vi "Seriell-ECD.vi"(0 "FPGA-VI-Referenz":refnum<k20>, 1 "SPvorgebenMod2":string[](array[string])=[":0622010121", ":0621010121", ":0626010121", ":0620010121", ":0624010121", ":0625010121", ":0623010121"], 5 "MWabfragenMod2":string[](array[string])=[":06220401210120", ":06210401210120", ":06260401210120", ":06200401210120", ":06240401210120", ":06250401210120", ":06230401210120"], 9 "MWAntwortMod2":string[](array[string])=[":0622020121", ":0621020121", ":0626020121", ":0620020121", ":0624020121", ":0625020121", ":0623020121"], 11 "FaktorMod2":dbl[](array[numeric])=[0.00625, 0.00625, 0.15625, 0.00015625, 0.00625, 0.00625, 0.00015625], 12 "SPquittieren":string[](array[string])=[":0422000005", ":0421000005", ":0426000005", ":0420000005", ":0424000005", ":0425000005", ":0423000005"]) -> (4 "Fehler":errorcluster)   [LabVIEW 2017]
uses:
  GVRefStrom.vi
  GVHorstSP.vi
  GVMWHorst.vi
  gvbooleschRT.vi
  <vilib>/Utility/error.llb/Error Cluster From Error Code.vi
  <vilib>/rvi/errors/niLvFpgaAdjustHostInterfaceError.vi
  GVECDs.vi
  <vilib>/rvi/interface/nirviMethod/nirviMethod.xnode
  FPGA Bitfiles/HAGAR-VECD_FPGATarget_FPGA-ProgrammECD_WS++LmW9gGg.lvbitx
  FPGA-Programm_ECD.vi
  <vilib>/regexp/Match Regular Expression.xnode
  <vilib>/FPGAPlugInAG/cRIO-9035/niLvFpga_WriteFifo_cRIO-9035.vi
  <vilib>/rvi/errors/niLvFpgaMergeErrorWithErrorCode.vi
  <vilib>/FPGAPlugInAG/cRIO-9035/niLvFpga_ReadFifo_cRIO-9035.vi
panel:
  in  "Fehler":errorcluster caption="Fehler (Ausgang)"
  out "ECD2":string
  out "ECD1":string
  out "Fehler":bool[](array[boolean])
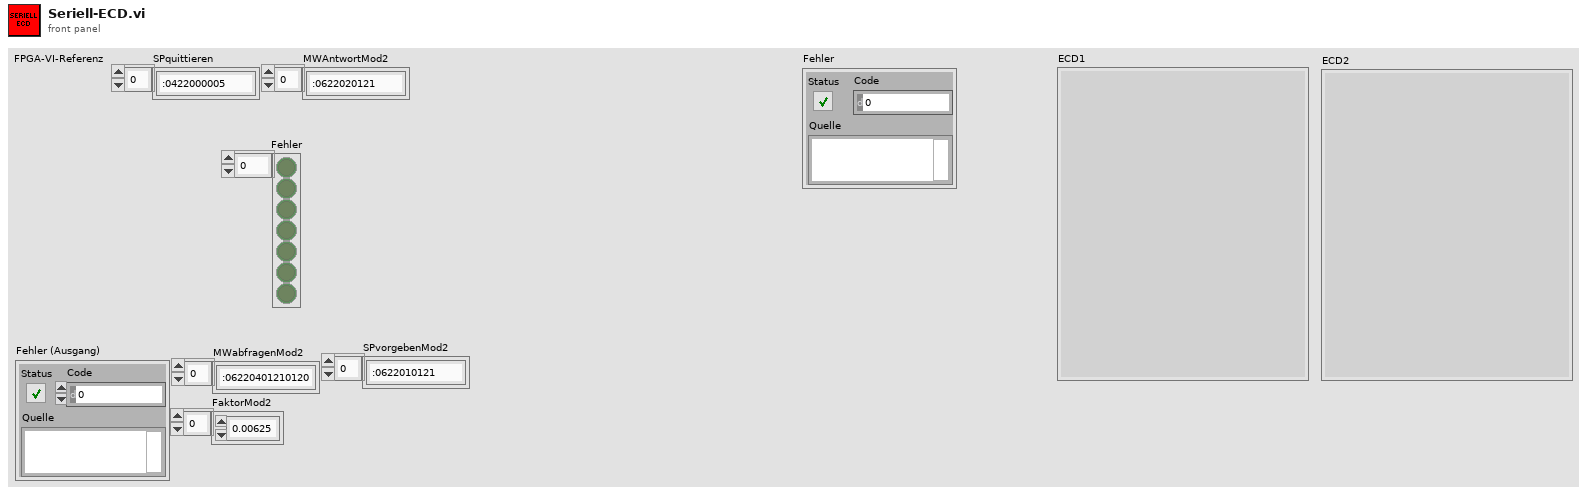
[diagram p1: front panel]
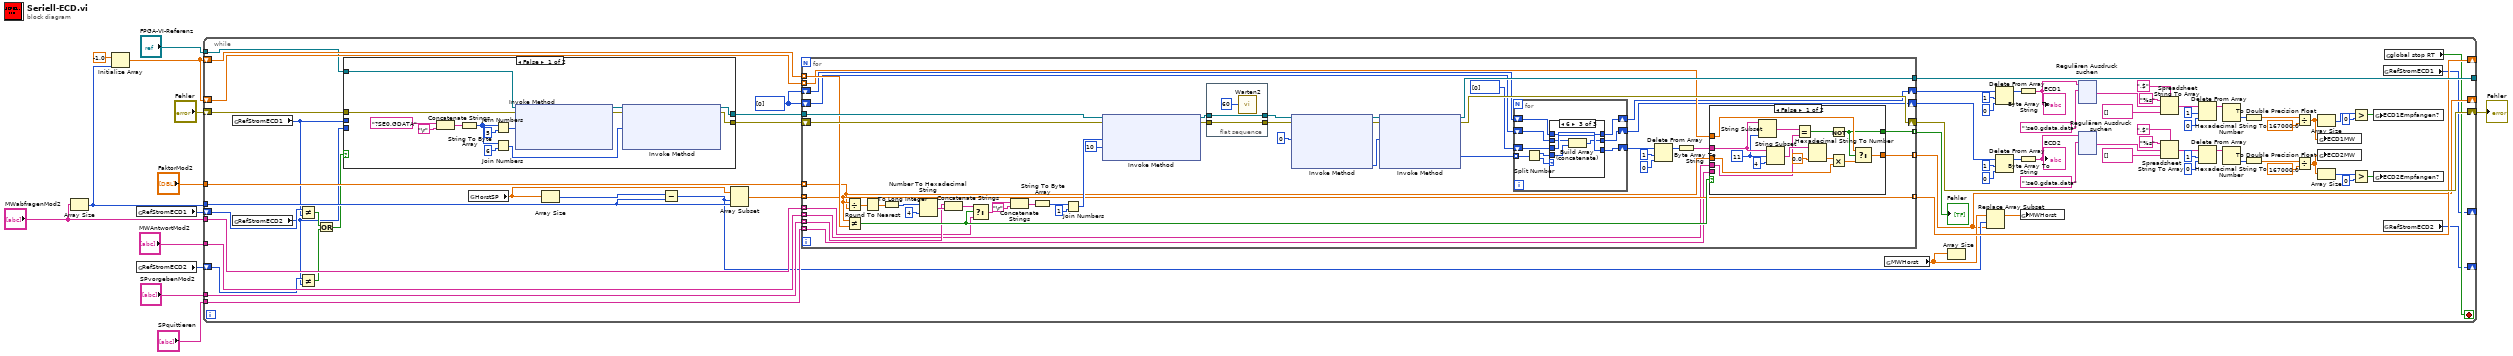
[diagram p0: block diagram]
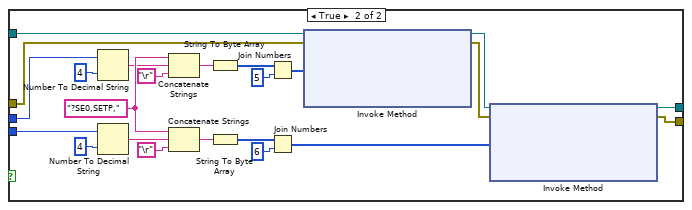
[diagram p2: hidden frame]
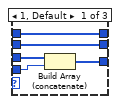
[diagram p3: hidden frame]
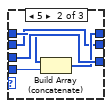
[diagram p4: hidden frame]
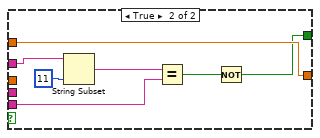
[diagram p5: hidden frame]
diagram:
  n1 = Array Size(array="MWabfragenMod2") -> (size(s)=w3:i32)
  n2 = Initialize Array(-1.0 ("Element"), w3) -> (w5:dbl[])
  n3 = global read "GVRefStrom.vi" "RefStromECD1"() -> (w2:i16)
  n4 = global read "GVRefStrom.vi" "RefStromECD2"() -> (w1:i16)
  n5 = while {
    shift-right: [w88] -> w4
    shift-left: "Fehler" -> [w68]
    shift-right: [w86] -> _
    shift-left: w5 -> [w87]
    shift-right: [w25] -> _
    shift-left: w5 -> [w84]
    tunnel: "SPvorgebenMod2" -> [w83]
    tunnel: "MWabfragenMod2" -> [w82]
    tunnel: "FaktorMod2" -> [w81]
    tunnel: "MWAntwortMod2" -> [w80]
    tunnel: "SPquittieren" -> [w79]
    tunnel: "FPGA-VI-Referenz" -> [w69]
    tunnel: [w89] -> _
    tunnel: w3 -> [w29]
    shift-right: [w22] -> _
    shift-left: w2 -> [w20]
    shift-right: [w21] -> _
    shift-left: w1 -> [w19]
    stop <- w23 stop-if-true
    w78 = u8[] [0]
    n6 = global read "GVRefStrom.vi" "RefStromECD1"() -> (w15:i16)
    n7 = global read "GVRefStrom.vi" "RefStromECD2"() -> (w14:i16)
    n8 = Not Equal?(x=w20, y=w15) -> (x != y?=w18:bool)
    n9 = Not Equal?(x=w19, y=w14) -> (x != y?=w17:bool)
    n10 = Or(x=w18, y=w17) -> (x .or. y?=w16:bool)
    n11 = case shown="False" w16 {
      tunnel: w69 -> [w103 w126]
      tunnel: w68 -> [w102 w125]
      tunnel: [w98 w121] -> w67
      tunnel: [w96 w119] -> w66
      tunnel: w15 -> [_ w105]
      tunnel: w14 -> [_ w104]
      frame False {
        n12 = Concatenate Strings("?SE0,GDATA" ("Schreibpuffer"), "\r") -> (w91:string)
        n13 = String To Byte Array(string=w91) -> (unsigned byte array=w90:u8[])
        n14 = Join Numbers(hi=w90, lo=u8 5) -> ((hi.lo)=w95:u16[])
        n15 = Join Numbers(hi=w90, lo=u8 6) -> ((hi.lo)=w94:u16[])
        n16 = xnode "Invoke Method"("FPGA-VI-Referenz (Eingang)"=w103, "Fehler (Eingang)"=w102, "Daten"=w95) -> ("FPGA-VI-Referenz (Ausgang)"=w99:refnum<k20>, "Fehler (Ausgang)"=w97:errorcluster)  [unwired: 1 in, 1 out]
        n17 = xnode "Invoke Method"("FPGA-VI-Referenz (Eingang)"=w99, "Fehler (Eingang)"=w97, "Daten"=w94) -> ("FPGA-VI-Referenz (Ausgang)"=w98:refnum<k20>, "Fehler (Ausgang)"=w96:errorcluster)  [unwired: 1 in, 1 out]
      }
      frame True {
        w110 = "?SE0,SETP," ("string")
        n18 = Number To Decimal String(number=w105, width (-)=i16 4) -> (decimal integer string=w109:string)
        n19 = Number To Decimal String(number=w104, width (-)=i16 4) -> (decimal integer string=w108:string)
        n20 = Concatenate Strings(w110, w109, "\r") -> (w115:string)
        n21 = Concatenate Strings(w110, w108, "\r") -> (w107:string)
        n22 = String To Byte Array(string=w115) -> (unsigned byte array=w114:u8[])
        n23 = String To Byte Array(string=w107) -> (unsigned byte array=w106:u8[])
        n24 = Join Numbers(hi=w114, lo=u8 5) -> ((hi.lo)=w118:u16[])
        n25 = Join Numbers(hi=w106, lo=u8 6) -> ((hi.lo)=w117:u16[])
        n26 = xnode "Invoke Method"("FPGA-VI-Referenz (Eingang)"=w126, "Fehler (Eingang)"=w125, "Daten"=w118) -> ("FPGA-VI-Referenz (Ausgang)"=w122:refnum<k20>, "Fehler (Ausgang)"=w120:errorcluster)  [unwired: 1 in, 1 out]
        n27 = xnode "Invoke Method"("FPGA-VI-Referenz (Eingang)"=w122, "Fehler (Eingang)"=w120, "Daten"=w117) -> ("FPGA-VI-Referenz (Ausgang)"=w121:refnum<k20>, "Fehler (Ausgang)"=w119:errorcluster)  [unwired: 1 in, 1 out]
      }
    }
    n28 = global read "GVHorstSP.vi" "HorstSP"() -> (w31:dbl[])
    n29 = Array Size(array=w31) -> (size(s)=w30:i32)
    n30 = Subtract(x=w30, y=w29) -> (x-y=w26:i32)
    n31 = Array Subset(array=w31, index=w26, length=w29) -> (w28:dbl[])
    n32 = for {
      tunnel: w87 -> [w370] mode=indexing
      tunnel: [w366] -> w86 mode=indexing
      tunnel: [w367] -> w85 mode=indexing
      shift-right: [w390] -> w88
      shift-left: w66 -> [w382]
      tunnel: w28 -> [w366] mode=indexing
      tunnel: w81 -> [w365] mode=indexing
      tunnel: [w364] -> w25 mode=indexing
      tunnel: w84 -> [w363] mode=indexing
      tunnel: w83 -> [w362] mode=indexing
      tunnel: w82 -> [w361] mode=indexing
      tunnel: w80 -> [w360] mode=indexing
      tunnel: w79 -> [w359] mode=indexing
      shift-right: [w349] -> w73
      shift-left: w78 -> [w352]
      shift-right: [w350] -> w72
      shift-left: w78 -> [w351]
      tunnel: w67 -> [w383]
      tunnel: [w393] -> w89
      n33 = Divide(x=w366, y=w365) -> (x/y=w377:dbl)
      n34 = Not Equal?(x=w366, y=w370) -> (x != y?=w368:bool)
      n35 = Round To Nearest(number=w377) -> (nearest integer value=w376:dbl)
      n36 = To Long Integer(number=w376) -> (32bit integer=w375:i32)
      n37 = Number To Hexadecimal String(1:i16 4 ("Breite (-)"), 2:w375) -> (0:w373:string)
      n38 = Concatenate Strings(w362, w373) -> (w372:string)
      n39 = Select(t=w372, s=w368, f=w361) -> (s? t:f=w371:string)
      n40 = Concatenate Strings(w371, "\r") -> (w389:string)
      n41 = String To Byte Array(string=w389) -> (unsigned byte array=w387:u8[])
      n42 = Join Numbers(hi=w387, lo=u8 1) -> ((hi.lo)=w388:u16[])
      n43 = xnode "Invoke Method"("FPGA-VI-Referenz (Eingang)"=w383, "Fehler (Eingang)"=w382, "Daten"=w388, "Timeout (ms)"=10) -> ("FPGA-VI-Referenz (Ausgang)"=w381:refnum<k20>, "Fehler (Ausgang)"=w379:errorcluster)  [unwired: 1 out]
      n44 = flat-sequence {
        tunnel: w381 -> [w443]
        tunnel: [w443] -> w380
        tunnel: w379 -> [w442]
        tunnel: [w442] -> w378
        frame #0 {
          n45 = call "Warten2"("Count(mSec)"=u32 60) -> ()  [unwired: 1 out]
        }
      }
      n46 = xnode "Invoke Method"("FPGA-VI-Referenz (Eingang)"=w380, "Fehler (Eingang)"=w378, "Anzahl der Elemente"=u32 0) -> ("FPGA-VI-Referenz (Ausgang)"=w392:refnum<k20>, "Fehler (Ausgang)"=w391:errorcluster, "Verbleibende Elemente"=w394:u32)  [unwired: 1 in, 1 out]
      n47 = xnode "Invoke Method"("FPGA-VI-Referenz (Eingang)"=w392, "Fehler (Eingang)"=w391, "Anzahl der Elemente"=w394) -> ("FPGA-VI-Referenz (Ausgang)"=w393:refnum<k20>, "Fehler (Ausgang)"=w390:errorcluster, "Daten"=w358:u16[])  [unwired: 1 in, 1 out]
      n48 = for {
        tunnel: w358 -> [w404] mode=indexing
        shift-right: [w398] -> w356
        shift-left: u8[] [0] -> [w399]
        shift-right: [w397] -> w349
        shift-left: w352 -> [w400]
        shift-right: [w396] -> w350
        shift-left: w351 -> [w401]
        n49 = Split Number(x=w404) -> (hi(x)=w402:u8, lo(x)=w403:u8)
        n50 = case shown="6" w403 {
          tunnel: w402 -> [w409 w412 w415]
          tunnel: w401 -> [w405 w410 w418]
          tunnel: w400 -> [w406 w413 w417]
          tunnel: w399 -> [w408 w414 w419]
          tunnel: [w407 w414 w419] -> w398
          tunnel: [w406 w411 w417] -> w397
          tunnel: [w405 w410 w416] -> w396
          frame 1, Default {
            n51 = Build Array (concatenate)(w408, w409) -> (w407:u8[])
          }
          frame 5 {
            n52 = Build Array (concatenate)(w413, w412) -> (w411:u8[])
          }
          frame 6 {
            n53 = Build Array (concatenate)(w418, w415) -> (w416:u8[])
          }
        }
      }
      n54 = Delete From Array(array=w356, length=1 ("Länge"), index=0 ("Index")) -> (array with subset deleted=w353:u8[])  [unwired: 1 out]
      n55 = Byte Array To String(unsigned byte array=w353) -> (string=w369:string)
      n56 = case shown="False" w368 {
        tunnel: w369 -> [w431 w440]
        tunnel: [w420 w434] -> w367
        tunnel: w365 -> [w425 _]
        tunnel: [w422 w436] -> w364
        tunnel: w363 -> [w423 w436]
        tunnel: w360 -> [w421 _]
        tunnel: w359 -> [_ w435]
        frame False {
          w430 = 11 ("Länge (Rest)")
          n57 = String Subset(string=w431, length (rest)=w430) -> (substring=w433:string)  [unwired: 1 in]
          n58 = String Subset(string=w431, offset (0)=w430, length (rest)=4 ("Länge (Rest)")) -> (substring=w428:string)
          n59 = Equal?(x=w433, y=w421) -> (x = y?=w432:bool)
          n60 = Hexadecimal String To Number(string=w428, default (0uL)=0.0 ("Standard (0 U32)")) -> (number=w426:dbl)  [unwired: 1 in, 1 out]
          n61 = Not(x=w432) -> (.not. x?=w420:bool)
          n62 = Multiply(x=w426, y=w425) -> (x*y=w424:dbl)
          n63 = Select(t=w423, s=w420, f=w424) -> (s? t:f=w422:dbl)
        }
        frame True {
          n64 = String Subset(string=w440, length (rest)=11 ("Länge (Rest)")) -> (substring=w439:string)  [unwired: 1 in]
          n65 = Equal?(x=w439, y=w435) -> (x = y?=w437:bool)
          n66 = Not(x=w437) -> (.not. x?=w434:bool)
        }
      }
    }
    "Fehler" <- w85
    n67 = global read "GVMWHorst.vi" "MWHorst"() -> (w27:dbl[])
    n68 = Array Size(array=w27) -> ()  [unwired: 1 out]
    n69 = Replace Array Subset(array=w27, new element=w25, index=w26) -> (w24:dbl[])
    n70 = Delete From Array(array=w73, length=1 ("Länge"), index=0 ("Index")) -> (array with subset deleted=w71:u8[])  [unwired: 1 out]
    n71 = Delete From Array(array=w72, length=1 ("Länge"), index=0 ("Index")) -> (array with subset deleted=w70:u8[])  [unwired: 1 out]
    n72 = Byte Array To String(unsigned byte array=w71) -> (string=w58:string)
    "ECD1" <- w58
    n73 = Byte Array To String(unsigned byte array=w70) -> (string=w40:string)
    "ECD2" <- w40
    n74 = global write "GVMWHorst.vi" "MWHorst"(w24) -> ()
    n75 = xnode "Regulären Ausdruck suchen"("Eingangs-String"=w58, "Regulärer Ausdruck"="!se0,gdata,data") -> ("Nach Übereinstimmung"=w59:string)  [unwired: 4 in, 4 out]
    n76 = xnode "Regulären Ausdruck suchen"("Eingangs-String"=w40, "Regulärer Ausdruck"="!se0,gdata,data") -> ("Nach Übereinstimmung"=w46:string)  [unwired: 4 in, 4 out]
    n77 = Spreadsheet String To Array(delimiter (Tab)=",$" ("Trennzeichen (Tabulator)"), format string="%s" ("Format-String"), spreadsheet string=w59, array type (2D Dbl)=string[] []) -> (array=w55:string[])
    n78 = Spreadsheet String To Array(delimiter (Tab)=",$" ("Trennzeichen (Tabulator)"), format string="%s" ("Format-String"), spreadsheet string=w46, array type (2D Dbl)=string[] []) -> (array=w43:string[])
    n79 = Delete From Array(array=w55, length=1 ("Länge"), index=0 ("Index")) -> (array with subset deleted=w53:string[])  [unwired: 1 out]
    n80 = Delete From Array(array=w43, length=1 ("Länge"), index=0 ("Index")) -> (array with subset deleted=w41:string[])  [unwired: 1 out]
    n81 = Hexadecimal String To Number(string=w53) -> (number=w62:u32[])  [unwired: 2 in, 1 out]
    n82 = Hexadecimal String To Number(string=w41) -> (number=w49:u32[])  [unwired: 2 in, 1 out]
    n83 = To Double Precision Float(number=w62) -> (double precision float=w61:dbl[])
    n84 = To Double Precision Float(number=w49) -> (double precision float=w48:dbl[])
    n85 = Divide(x=w61, y=167000.0) -> (x/y=w39:dbl[])
    n86 = Divide(x=w48, y=167000.0) -> (x/y=w33:dbl[])
    n87 = Array Size(array=w39) -> (size(s)=w38:i32)
    n88 = global write "GVECDs.vi" "ECD1MW"(w39) -> ()
    n89 = global write "GVECDs.vi" "ECD2MW"(w33) -> ()
    n90 = Array Size(array=w33) -> (size(s)=w35:i32)
    n91 = Greater?(x=w38, y=0) -> (0:w36:bool)
    n92 = Greater?(x=w35, y=0) -> (0:w32:bool)
    n93 = global write "GVECDs.vi" "ECD1Empfangen?"(w36) -> ()
    n94 = global write "GVECDs.vi" "ECD2Empfangen?"(w32) -> ()
    n95 = global read "GVRefStrom.vi" "RefStromECD1"() -> (w22:i16)
    n96 = global read "GVRefStrom.vi" "RefStromECD2"() -> (w21:i16)
    n97 = global read "gvbooleschRT.vi" "global stop RT"() -> (w23:bool)
  }
  "Fehler" <- w4
